vi "clear HASO4_3 timeout error.vi"(8 "error in (no error)":errorcluster) -> (0 "error out":errorcluster)   [LabVIEW 2020, in "HASO4_3.lvclass"]
uses:
  HASO4_3.lvclass
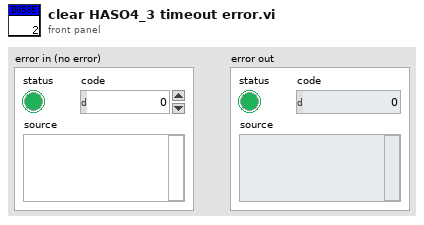
[diagram p1: front panel]
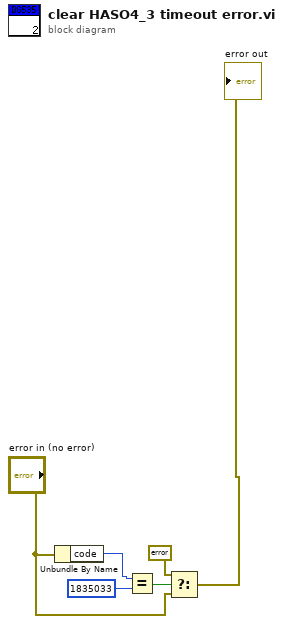
[diagram p0: block diagram]
diagram:
  n1 = Unbundle By Name("error in (no error)") -> ("code"=w3:i32)
  n2 = Equal?(x=w3, y=1835033) -> (x = y?=w1:bool)
  n3 = Select(t=errorcluster {"status"=FALSE, "code"=0, "source"=""} ("error out"), s=w1, f="error in (no error)") -> (s? t:f=→"error out":errorcluster)
